vi "meshgrid.vi"(10 "Y in":dbl[](array[numeric]), 11 "X in":dbl[](array[numeric])) -> (2 "Y":dbl[][](array[numeric]), 3 "X":dbl[][](array[numeric]))   [LabVIEW 2022 SP3]
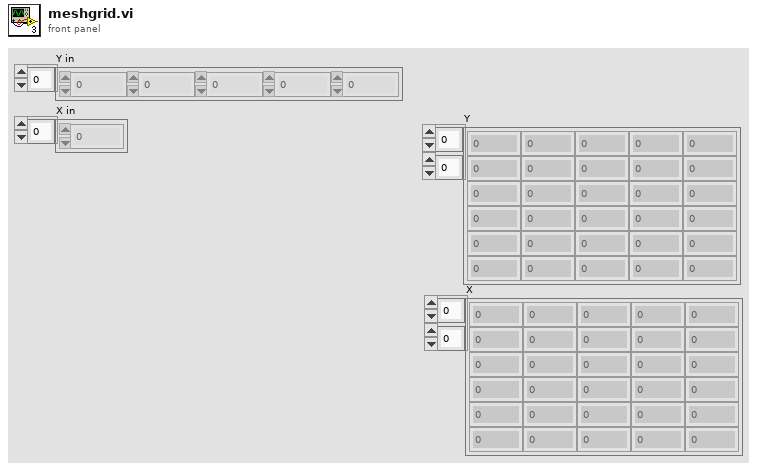
[diagram p1: front panel]
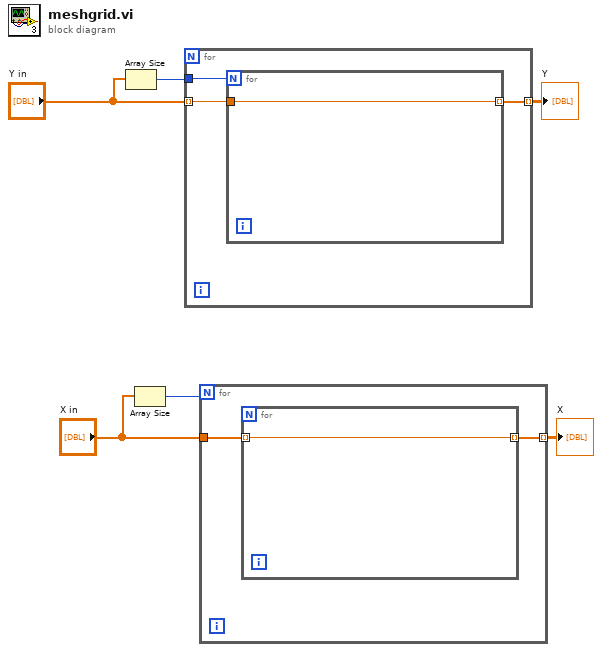
[diagram p0: block diagram]
diagram:
  n1 = Array Size(array="Y in") -> (size(s)=w6:i32)
  n2 = Array Size(array="X in") -> (size(s)=w3:i32)
  n3 = for {
    tunnel: "Y in" -> [w9] mode=indexing
    tunnel: w6 -> [w8]
    tunnel: [w7] -> w5 mode=indexing
    n4 = for {
      N: w8 -> [_]
      tunnel: w9 -> [w10]
      tunnel: [w10] -> w7 mode=indexing
    }
  }
  "Y" <- w5
  n5 = for {
    N: w3 -> [_]
    tunnel: "X in" -> [w12]
    tunnel: [w11] -> w4 mode=indexing
    n6 = for {
      tunnel: w12 -> [w13] mode=indexing
      tunnel: [w13] -> w11 mode=indexing
    }
  }
  "X" <- w4
